vi "GetDiagramInputs.vi"(6 "error in":errorcluster, 9 "FlatSequenceFrame in":refnum<class "FlatSequenceFrame.lvclass">) -> (0 "error out":errorcluster, 3 "FlatSequenceFrame out":refnum<class "FlatSequenceFrame.lvclass">, 4 "inputs terminals":refnum<class "Terminal.lvclass">[][](array[class]))   [LabVIEW 2014, in "FlatSequenceFrame.lvclass"]
uses:
  FlatSequenceFrame.lvclass
  Terminal/Terminal.lvclass
  FlatSequenceFrame.lvclass/FlatSequenceFrame.ctl
  FlatSequenceInnerTunnel/FlatSequenceInnerTunnel.lvclass/FlatSequenceInnerTunnel.ctl
  FlatSequenceOuterTunnel/FlatSequenceOuterTunnel.lvclass/FlatSequenceOuterTunnel.ctl
  FlatSequenceInnerTunnel/FlatSequenceInnerTunnel.lvclass
  FlatSequenceOuterTunnel/FlatSequenceOuterTunnel.lvclass
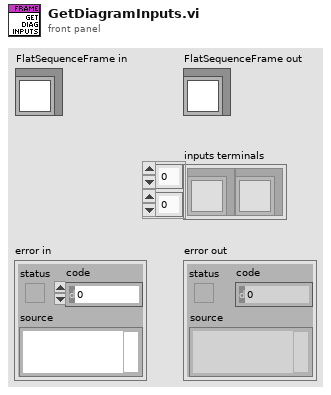
[diagram p1: front panel]
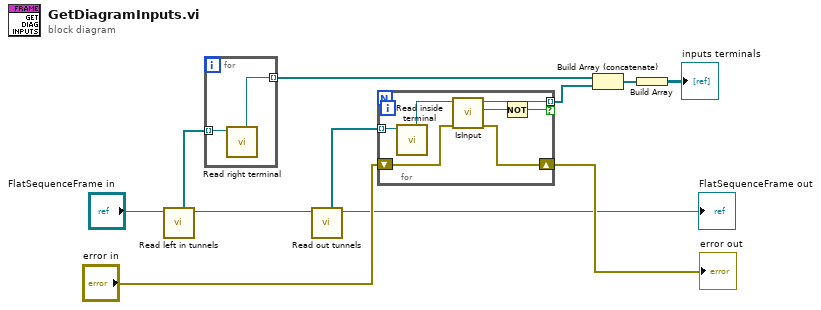
[diagram p0: block diagram]
diagram:
  n1 = call "Read left in tunnels.vi"("FlatSequenceFrame in"="FlatSequenceFrame in") -> ("FlatSequenceFrame out"=w9:refnum<class "FlatSequenceFrame.lvclass">, "left in tunnels"=w10:refnum<class "FlatSequenceInnerTunnel.lvclass">[])  [unwired: 7 in]
  n2 = for {
    tunnel: w10 -> [w13] mode=indexing
    tunnel: [w12] -> w7 mode=indexing
    n3 = call "Read right terminal.vi"("FlatSequenceInnerTunnel in"=w13) -> ("right terminal"=w12:refnum<class "Terminal.lvclass">)  [unwired: 7 in, 1 out]
  }
  n4 = call "Read out tunnels.vi"("FlatSequenceFrame in"=w9) -> ("FlatSequenceFrame out"=→"FlatSequenceFrame out":refnum<class "FlatSequenceFrame.lvclass">, "out tunnels"=w8:refnum<class "FlatSequenceOuterTunnel.lvclass">[])  [unwired: 7 in]
  n5 = for {
    tunnel: w8 -> [w20] mode=indexing
    tunnel: [w18] -> w6 mode=indexing if=w14
    shift-right: [w16] -> w2
    shift-left: "error in" -> [w17]
    n6 = call "Read inside terminal.vi"("FlatSequenceInnerTunnel in"=w20) -> ("inside terminal"=w19:refnum<class "Terminal.lvclass">)  [unwired: 7 in, 1 out]
    n7 = call-dynamic "IsInput.vi"("error in"=w17, "Terminal in"=w19) -> ("error out"=w16:errorcluster, "input"=w15:bool, "Terminal out"=w18:refnum<class "Terminal.lvclass">)  [unwired: 5 in]
    n8 = Not(x=w15) -> (.not. x?=w14:bool)
  }
  "error out" <- w2
  n9 = Build Array (concatenate)(w7, w6) -> (w5:refnum<class "Terminal.lvclass">[])
  n10 = Build Array(w5) -> (→"inputs terminals":refnum<class "Terminal.lvclass">[][])
